vi "Graphic_Interface.vi"() -> ()   [LabVIEW 2013]
uses:
  <vilib>/Instr/_visa.llb/VISA Configure Serial Port (Instr).vi
panel:
  out "Numeric 4":dbl
  out "Numeric 3":dbl
  out "Numeric 2":dbl
  out "Numeric":dbl
  out "Pot01":dbl(knob) scale=0.0..5.0
  out "String 4":string
  out "String 3":string
  out "String 2":string
  out "String":string
  out "Pot02":dbl(slide) scale=0.0..5.0
  out "Pot04":dbl(knob) scale=0.0..5.0
  out "Pot03":dbl(slide) scale=0.0..5.0
  out "read buffer":string
  in  "Puerto COM:":refnum<visa-resource-name>
  in  "stop":bool
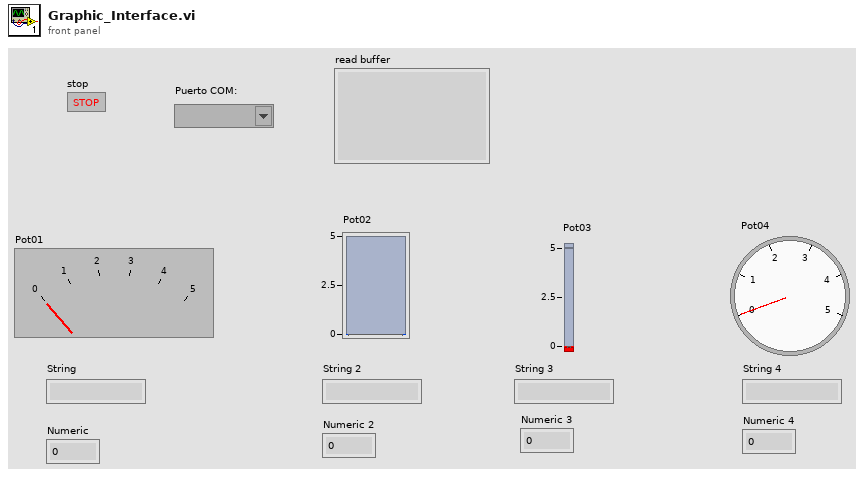
[diagram p1: front panel]
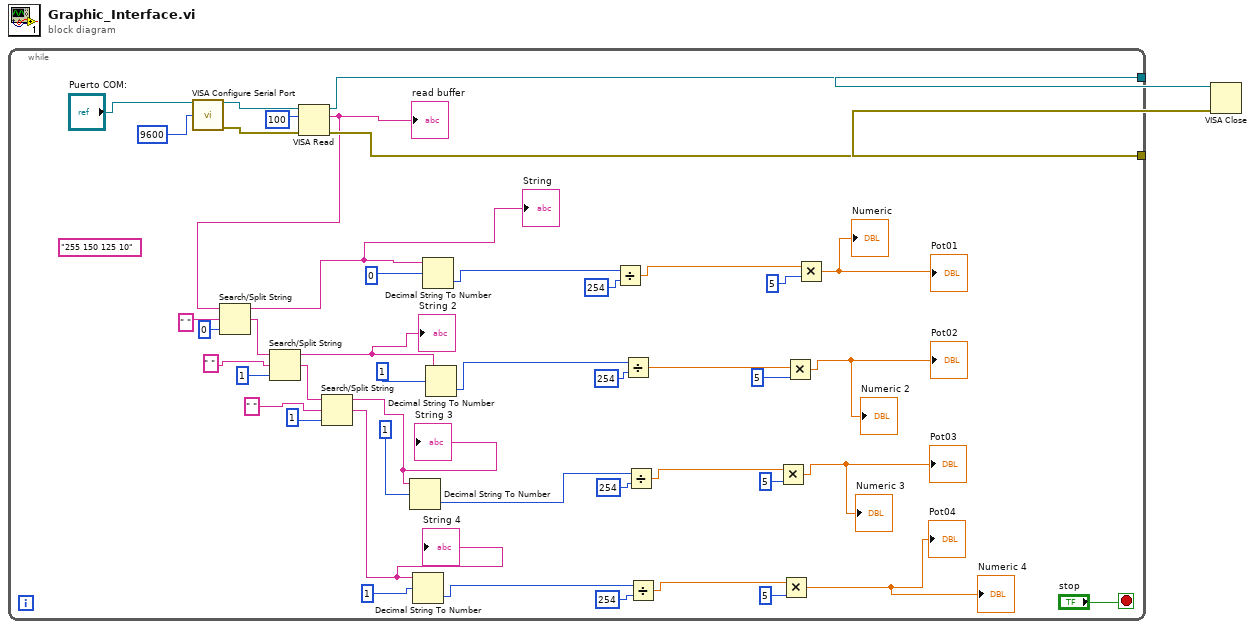
[diagram p0: block diagram]
diagram:
  n1 = while {
    tunnel: [w4] -> w2
    tunnel: [w43] -> w1
    stop <- "stop" stop-if-true
    (unwired) "255 150 125 10"
    n2 = call-poly "VISA Configure Serial Port"("VISA resource name"="Puerto COM:", "data bits (8)"=9600) -> ("VISA resource name out"=w5:refnum<visa-resource-name>, "error out"=w45:errorcluster)  [unwired: 12 in]
    n3 = VISA Read(VISA resource name=w5, byte count=u32 100, error in (no error)=w45) -> (VISA resource name out=w4:refnum<visa-resource-name>, read buffer=w6:string, error out=w43:errorcluster)  [unwired: 1 out]
    "read buffer" <- w6
    n4 = Search/Split String(string=w6, search string/char (-)=" ", offset (0)=0) -> (substring before match=w32:string, match + rest of string=w42:string)  [unwired: 1 out]
    "String" <- w32
    n5 = Search/Split String(string=w42, search string/char (-)=" ", offset (0)=1) -> (substring before match=w31:string, match + rest of string=w41:string)  [unwired: 1 out]
    "String 2" <- w31
    n6 = Search/Split String(string=w41, search string/char (-)=" ", offset (0)=1) -> (substring before match=w30:string, match + rest of string=w29:string)  [unwired: 1 out]
    "String 3" <- w30
    "String 4" <- w29
    n7 = Decimal String To Number(string=w30, offset=1) -> (number=w16:i32)  [unwired: 1 in, 1 out]
    n8 = Decimal String To Number(string=w29, offset=1) -> (number=w15:i32)  [unwired: 1 in, 1 out]
    n9 = Decimal String To Number(string=w32, offset=0) -> (number=w18:i32)  [unwired: 1 in, 1 out]
    n10 = Decimal String To Number(string=w31, offset=1) -> (number=w17:i32)  [unwired: 1 in, 1 out]
    n11 = Divide(x=w18, y=254) -> (x/y=w26:dbl)
    n12 = Divide(x=w17, y=254) -> (x/y=w25:dbl)
    n13 = Divide(x=w16, y=254) -> (x/y=w24:dbl)
    n14 = Divide(x=w15, y=254) -> (x/y=w23:dbl)
    n15 = Multiply(x=w24, y=5) -> (x*y=→"Pot03" →"Numeric 3":dbl)
    n16 = Multiply(x=w23, y=5) -> (x*y=→"Pot04" →"Numeric 4":dbl)
    n17 = Multiply(x=w25, y=5) -> (x*y=→"Pot02" →"Numeric 2":dbl)
    n18 = Multiply(x=w26, y=5) -> (x*y=→"Pot01" →"Numeric":dbl)
  }
  n19 = VISA Close(VISA resource name=w2, error in (no error)=w1) -> ()  [unwired: 1 out]
